vi "Config DispSnsr.vi"(8 "error in (no error)":errorcluster, 11 "Configuration in":refnum<class "Configuration.lvclass">) -> (0 "error out":errorcluster, 3 "Configuration out":refnum<class "Configuration.lvclass">)   [LabVIEW 2016, in "Hardware.lvlib" / "Displacement Sensor.lvlib" / "DispSnsr Configuration.lvclass"]
uses:
  <userlib>/Common Components/Hardware/Displacement Sensor/DispSnsr Config/DispSnsr Configuration.lvclass
  <userlib>/Configuration Dialog Actor/Configuration.lvclass
  C:/Program Files (x86)/National Instruments/LabVIEW 2016/user.lib/Configuration Dialog Actor/Configuration.lvclass
  <userlib>/Common Components/Hardware/Displacement Sensor/DispSnsr Config/DispSnsr Configuration.lvclass/DispSnsr Configuration.ctl
  <userlib>/Common Components/Hardware/Abstract Hardware/Hardware.lvclass/Hardware.ctl
  <userlib>/Common Components/Hardware/DevInfo/DevInfo.lvclass/DevInfo.ctl
  <userlib>/Common Components/Hardware/Abstract Hardware/Read DevInfo.vi
  <userlib>/Common Components/Hardware/DevInfo/Read COMM Address.vi
  <userlib>/Common Components/Hardware/DevInfo/Read Sub-COMM Address.vi
  <userlib>/Common Components/Hardware/DevInfo/Read HW Type.vi
  <userlib>/Common Components/Hardware/DevInfo/Read Device Name.vi
  <userlib>/Common Components/Hardware/DevInfo/Read Status.vi
  <userlib>/Common Components/Hardware/Displacement Sensor/DispSnsr/DispSnsr.lvclass
  C:/Program Files (x86)/National Instruments/LabVIEW 2016/user.lib/Common Components/Hardware/Abstract Hardware/Hardware.lvclass
  <userlib>/Common Components/Hardware/DevInfo/DevInfo.lvclass
panel:
  out "Status":bool
  out "HW Type":string
  out "Sub-COMM Address":string
  out "COMM Address":string
  out "Device Name":string
  in  "Revert":bool
  in  "Apply":bool
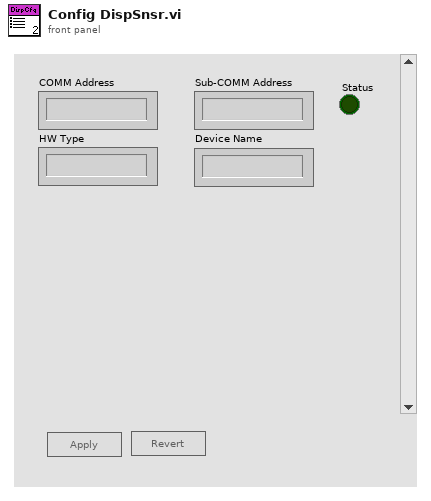
[diagram p1: front panel]
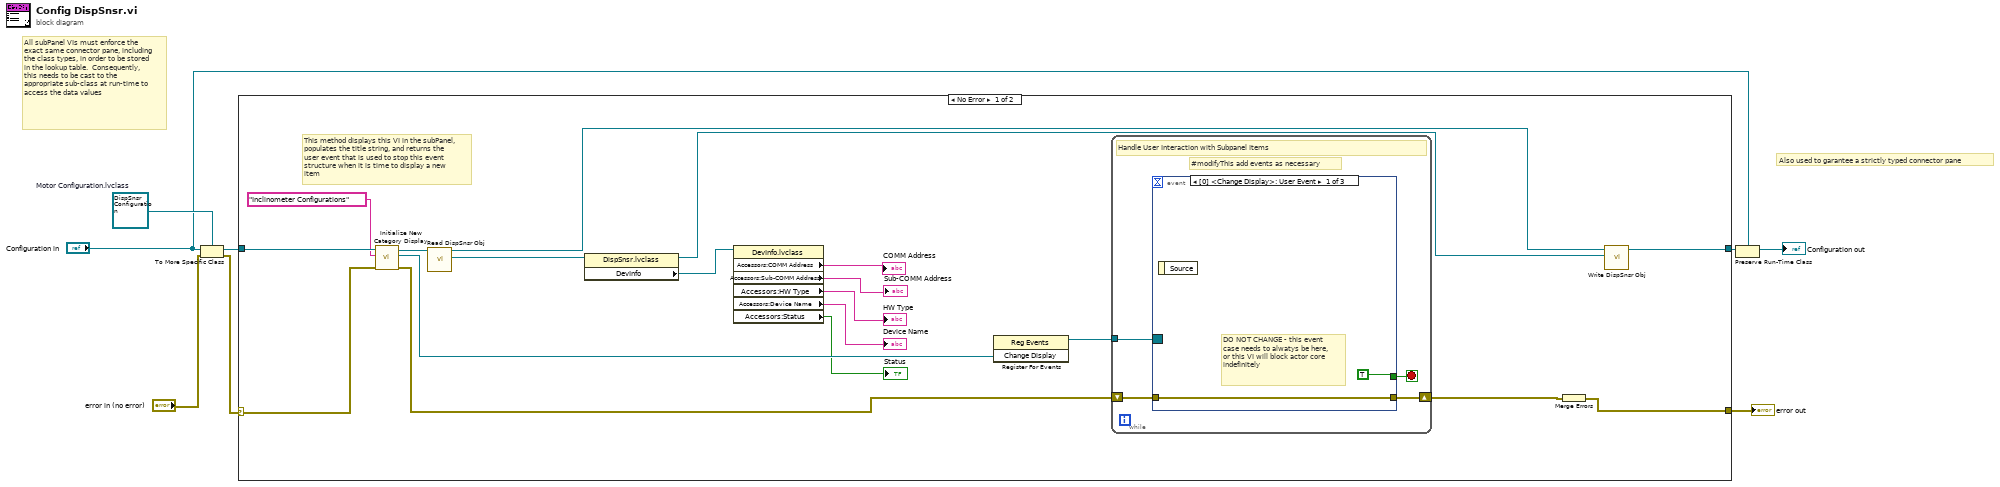
[diagram p0: block diagram]
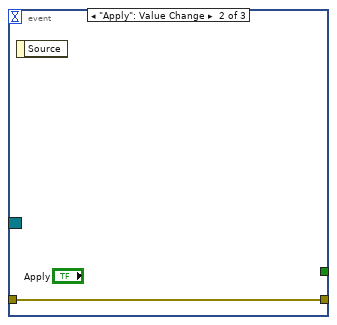
[diagram p2: hidden frame]
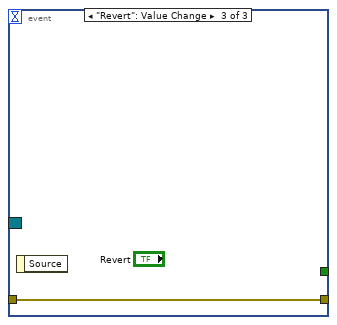
[diagram p3: hidden frame]
diagram:
  w5 = refnum<class "DispSnsr Configuration.lvclass"> refnum  # Motor Configuration.lvclass
  # "Also used to garantee a strictly typed connector pane"
  # "All subPanel VIs must enforce the exact same connector pane, including the class types, in order to be stored in the lookup table.  Consequently, this needs to be cast to the appropriate sub-class at run-time to access the data values"
  n1 = To More Specific Class(target class=w5, reference="Configuration in", error in="error in (no error)") -> (specific class reference=w6:refnum<class "DispSnsr Configuration.lvclass">, error out=w1:errorcluster)
  n2 = case shown="No Error" w1 {
    selector: w1 -> [w22 w36]
    tunnel: w6 -> [w27 w37]
    tunnel: [w11 w37] -> w8
    tunnel: [w24 w36] -> w7
    frame No Error {
      # "This method displays this VI in the subPanel, populates the title string, and returns the user event that is used to stop this event structure when it is time to display a new item"
      n3 = call <userlib>:"Initialize New Category Display.vi"("error in (no error)"=w22, "Name to Display"="Inclinometer Configurations", "Configuration in"=w27) -> ("error out"=w25:errorcluster, "Change Display"=w21:refnum<user-event>, "Configuration Out"=w26:refnum<class "DispSnsr Configuration.lvclass">)  [unwired: 6 in]
      n4 = call <userlib>:"Read DispSnsr Obj.vi"("DispSnsr Configuration in"=w26) -> ("Hardware.lvlib:Displacement Sensor.lvlib:DispSnsr.lvclass"=w15:refnum<class "DispSnsr.lvclass">, "DispSnsr Configuration out"=w10:refnum<class "DispSnsr Configuration.lvclass">)  [unwired: 9 in]
      n5 = property class="DispSnsr.lvclass"(reference=w15) -> (reference out=w9:refnum<class "DispSnsr.lvclass">, "DevInfo"=w14:refnum<class "DevInfo.lvclass">)  [unwired: 1 in, 1 out]
      n6 = property class="DevInfo.lvclass"(reference=w14) -> ("Accessors:COMM Address"=→"COMM Address":string, "Accessors:Sub-COMM Address"=→"Sub-COMM Address":string, "Accessors:HW Type"=→"HW Type":string, "Accessors:Device Name"=→"Device Name":string, "Accessors:Status"=→"Status":bool)  [unwired: 1 in, 2 out]
      n7 = register-events(w21) -> (reference out=w13:refnum<event-registration>)  [unwired: 2 in, 1 out]
      n8 = while {
        tunnel: w13 -> [w30]
        shift-right: [w29] -> w12
        shift-left: w25 -> [w28]
        stop <- w31 stop-if-true
        # "#modifyThis add events as necessary"
        # "Handle User Interaction with Subpanel Items"
        n9 = event shown="[0] <Change Display>: User Event" {
          selector: w30 -> [_ _ _]
          dyn-events: _ -> [_ _ _]
          timeout: _ -> [_ _ _]
          tunnel: [TRUE _ _] -> w31
          tunnel: [w32 w34 w35] -> w29
          tunnel: w28 -> [w32 w34 w35]
          event User Event {
            # "DO NOT CHANGE - this event case needs to alwatys be here, or this VI will block actor core indefinitely"
            n10 = event-data() -> ()  [unwired: 1 in, 1 out]
          }
          event "Apply": Value Change {
            n11 = event-data() -> ()  [unwired: 1 in, 1 out]
          }
          event "Revert": Value Change {
            n12 = event-data() -> ()  [unwired: 1 in, 1 out]
          }
        }
      }
      n13 = Merge Errors(w12) -> (w24:errorcluster)
      n14 = call <userlib>:"Write DispSnsr Obj.vi"("Hardware.lvlib:Displacement Sensor.lvlib:DispSnsr.lvclass"=w9, "DispSnsr Configuration in"=w10) -> ("DispSnsr Configuration out"=w11:refnum<class "DispSnsr Configuration.lvclass">)  [unwired: 9 in]
    }
    frame Error {
    }
  }
  "error out" <- w7
  n15 = Preserve Run-Time Class(object in=w8, 2:"Configuration in") -> (object out=→"Configuration out":refnum<class "Configuration.lvclass">)  [unwired: 1 in, 1 out]
